vi "波形发生器.vi"(3 "sampling info":cluster{"Fs":dbl, "#s":dbl}={"Fs"=1000.0, "#s"=1000.0} caption="采样信息" {"Fs" format="%.2p"}, 4 "formula":string="sin(w*t)*sin(2*pi(1)*t)" caption="公式", 5 "duty cycle (%)":dbl=50.0 caption="占空比(%)" format="%0.2f", 6 "phase":dbl caption="相位" format="%.2p", 7 "amplitude":dbl=1.0 caption="幅值" format="%0.2p", 8 "frequency":dbl=10.0 caption="频率" format="%0.2p", 9 "信噪比":dbl, 10 "噪声选择":enum16{"无", "均匀白噪声"}(ring), 11 "波形选择":enum16{"正弦波", "方波", "三角波", "公式波形"}(ring)) -> (1 "波形图":waveform(dbl)(graph))   [LabVIEW 2017]
uses:
  <vilib>/measure/NI_MABase.lvlib
  <vilib>/measure/NI_MAPro.lvlib
panel:
  # "波形发生器"
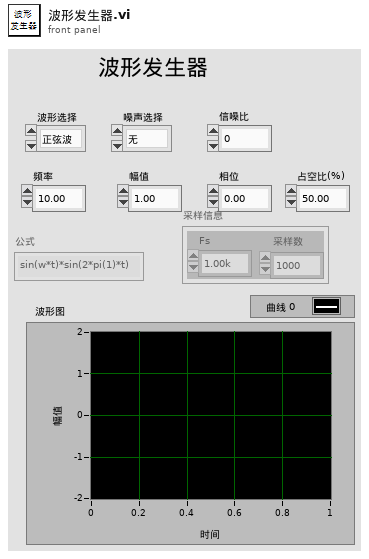
[diagram p1: front panel]
types:
  T1 = enum8{"Enabled", "Disabled", "Disabled and Grayed Out"}
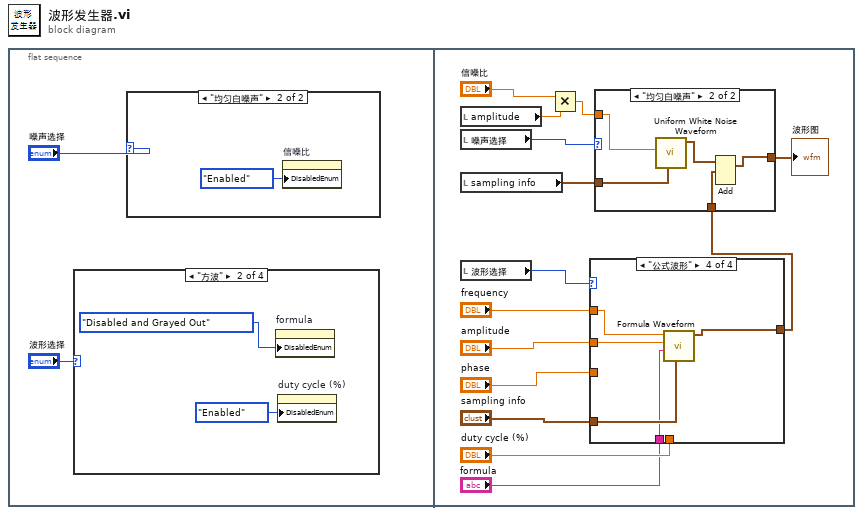
[diagram p0: block diagram]
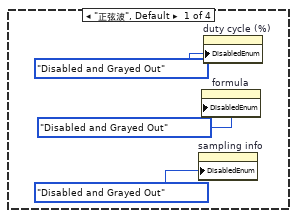
[diagram p2: hidden frame]
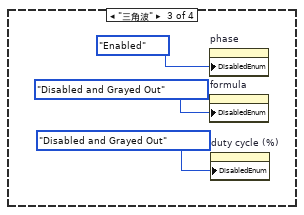
[diagram p3: hidden frame]
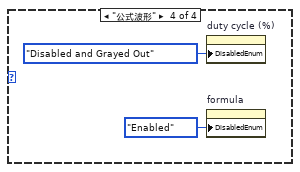
[diagram p4: hidden frame]
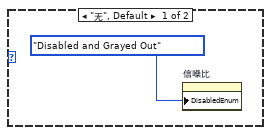
[diagram p5: hidden frame]
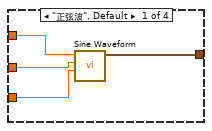
[diagram p7: hidden frame]
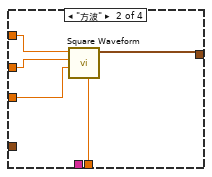
[diagram p8: hidden frame]
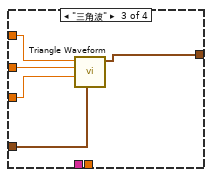
[diagram p9: hidden frame]
diagram:
  n1 = flat-sequence {
    frame #0 {
      n2 = case shown="\"方波\"" "波形选择" {
        frame "正弦波", Default {
          n3 = property on="sampling info" class="Clust (严格)"("DisabledEnum"=T1."Disabled and Grayed Out" ("禁用")) -> ()  [unwired: 2 in, 2 out]
          n4 = property on="formula" class="Str"("DisabledEnum"=T1."Disabled and Grayed Out" ("禁用")) -> ()  [unwired: 2 in, 2 out]
          n5 = property on="duty cycle (%)" class="DigNum (严格)"("DisabledEnum"=T1."Disabled and Grayed Out" ("禁用")) -> ()  [unwired: 2 in, 2 out]
        }
        frame "方波" {
          n6 = property on="formula" class="Str"("DisabledEnum"=T1."Disabled and Grayed Out" ("禁用")) -> ()  [unwired: 2 in, 2 out]
          n7 = property on="duty cycle (%)" class="DigNum (严格)"("DisabledEnum"=T1."Enabled" ("禁用")) -> ()  [unwired: 2 in, 2 out]
        }
        frame "三角波" {
          n8 = property on="phase" class="DigNum (严格)"("DisabledEnum"=T1."Enabled" ("禁用")) -> ()  [unwired: 2 in, 2 out]
          n9 = property on="formula" class="Str"("DisabledEnum"=T1."Disabled and Grayed Out" ("禁用")) -> ()  [unwired: 2 in, 2 out]
          n10 = property on="duty cycle (%)" class="DigNum (严格)"("DisabledEnum"=T1."Disabled and Grayed Out" ("禁用")) -> ()  [unwired: 2 in, 2 out]
        }
        frame "公式波形" {
          n11 = property on="duty cycle (%)" class="DigNum (严格)"("DisabledEnum"=T1."Disabled and Grayed Out" ("禁用")) -> ()  [unwired: 2 in, 2 out]
          n12 = property on="formula" class="Str"("DisabledEnum"=T1."Enabled" ("禁用")) -> ()  [unwired: 2 in, 2 out]
        }
      }
      n13 = case shown="\"均匀白噪声\"" "噪声选择" {
        frame "无", Default {
          n14 = property on="信噪比" class="DigNum (严格)"("DisabledEnum"=T1."Disabled and Grayed Out" ("禁用")) -> ()  [unwired: 2 in, 2 out]
        }
        frame "均匀白噪声" {
          n15 = property on="信噪比" class="DigNum (严格)"("DisabledEnum"=T1."Enabled" ("禁用")) -> ()  [unwired: 2 in, 2 out]
        }
      }
    }
    frame #1 {
      n16 = local read "amplitude"() -> (w19:dbl)
      n17 = local read "噪声选择"() -> (w21:enum16{"无", "均匀白噪声"})
      n18 = local read "sampling info"() -> (w17:cluster{"Fs":dbl, "#s":dbl})
      n19 = local read "波形选择"() -> (w28:enum16{"正弦波", "方波", "三角波", "公式波形"})
      n20 = Multiply(x="信噪比", y=w19) -> (x*y=w18:dbl)
      n21 = case shown="\"公式波形\"" w28 {
        tunnel: "frequency" -> [w38 w43 w48 w53]
        tunnel: "amplitude" -> [w37 w42 w47 w52]
        tunnel: "phase" -> [w36 w41 w46 _]
        tunnel: "sampling info" -> [_ _ w45 w51]
        tunnel: "duty cycle (%)" -> [_ w40 _ _]
        tunnel: "formula" -> [_ _ _ w50]
        tunnel: [w35 w39 w44 w49] -> w16
        frame "正弦波", Default {
          n22 = call <vilib>:"Sine Waveform.vi"("phase"=w36, "amplitude"=w37, "frequency"=w38) -> ("signal out"=w35:waveform(dbl))  [unwired: 7 in, 1 out]
        }
        frame "方波" {
          n23 = call <vilib>:"Square Waveform.vi"("duty cycle (%)"=w40, "phase"=w41, "amplitude"=w42, "frequency"=w43) -> ("signal out"=w39:waveform(dbl))  [unwired: 6 in, 1 out]
        }
        frame "三角波" {
          n24 = call <vilib>:"Triangle Waveform.vi"("sampling info"=w45, "phase"=w46, "amplitude"=w47, "frequency"=w48) -> ("signal out"=w44:waveform(dbl))  [unwired: 6 in, 1 out]
        }
        frame "公式波形" {
          n25 = call <vilib>:"Formula Waveform.vi"("sampling info"=w51, "formula"=w50, "amplitude"=w52, "frequency"=w53) -> ("signal out"=w49:waveform(dbl))  [unwired: 6 in, 1 out]
        }
      }
      n26 = case shown="\"均匀白噪声\"" w21 {
        tunnel: w18 -> [_ w34]
        tunnel: w17 -> [_ w33]
        tunnel: w16 -> [w29 w32]
        tunnel: [w29 w30] -> w15
        frame "无", Default {
        }
        frame "均匀白噪声" {
          n27 = call <vilib>:"Uniform White Noise Waveform.vi"("sampling info"=w33, "seed"=w34) -> ("signal out"=w31:waveform(dbl))  [unwired: 8 in, 1 out]
          n28 = Add(1:w32, 2:w31) -> (0:w30:waveform(dbl))  [unwired: 1 in, 1 out]
        }
      }
      "波形图" <- w15
    }
  }
